vi "SetAuto0.vi"(8 "Temp Ambiant":dbl, 11 "Longueur d'onde":dbl) -> (2 "0 à température ambiante":dbl)   [LabVIEW 2018]
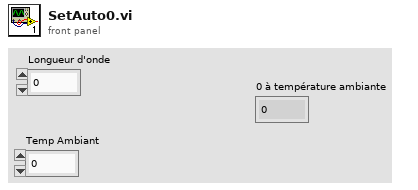
[diagram p1: front panel]
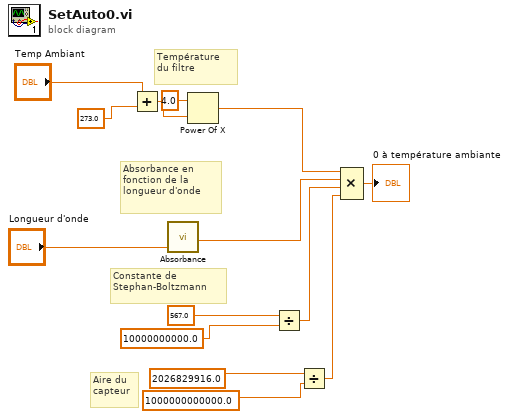
[diagram p0: block diagram]
diagram:
  # "Constante de \nStephan-Boltzmann"
  # "Absorbance en\nfonction de la \nlongueur d'onde"
  # "Température \ndu filtre"
  # "Aire du\ncapteur"
  n1 = Add(x="Temp Ambiant", y=273.0) -> (x+y=w14:dbl)
  n2 = call "Absorbance.vi"("Longueur d'onde"="Longueur d'onde") -> ("absorbance"=w6:dbl)  [unwired: 10 in]
  n3 = Power Of X(1:w14, 2:4.0 ("y")) -> (0:w5:dbl)
  n4 = Divide(x=567.0, y=10000000000.0) -> (x/y=w7:dbl)
  n5 = Divide(x=2026829916.0, y=1000000000000.0) -> (x/y=w8:dbl)
  n6 = Compound Arithmetic op=MULTIPLY(w5, w6, w7, w8) -> (→"0 à température ambiante":dbl)
